vi "Send Launch Models.vi"(8 "error in (no error)":errorcluster, 11 "Message Enqueuer in":refnum<class "Message Enqueuer.lvclass">) -> (0 "error out":errorcluster, 3 "Message Enqueuer out":refnum<class "Message Enqueuer.lvclass">)   [LabVIEW 2015, in "UI Controller.lvlib"]
uses:
  UI Controller.lvlib
  <vilib>/ActorFramework/Message Enqueuer/Message Enqueuer.lvclass
  Models/Settings Model/Settings Model/Settings Model.lvclass
  Models/Message Dialog Model/Message Dialog Model/Message Dialog Model.lvclass
  Models/Print Model/Print Model/Print Model.lvclass
  Hide Subpanel Msg/Hide Subpanel Msg.lvclass
  Hide Subpanel Msg/Hide Subpanel Msg.lvclass/Hide Subpanel Msg.ctl
  <vilib>/ActorFrameworkMVC/Abstract Controller/Abstract Controller Messages/Launch Model Msg/Launch Model Msg.lvclass/Launch Model Msg.ctl
  <vilib>/ActorFramework/Message Enqueuer/Message Enqueuer.lvclass/Message Enqueuer.ctl
  <vilib>/ActorFramework/Self-Addressed Msg/Self-Addressed Msg.lvclass/Self-Addressed Msg.ctl
  Models/Print Model/Print Model/Print Model.lvclass/Print Model.ctl
  <vilib>/ActorFramework/Message Enqueuer/Enqueue.vi
  <vilib>/ActorFramework/Message Priority Queue/Priority Enqueue.vi
  <vilib>/ActorFrameworkMVC/Abstract Controller/Abstract Controller Messages/Launch Model Msg/Launch Model Msg.lvclass
  <vilib>/ActorFramework/Self-Addressed Msg/Self-Addressed Msg.lvclass
panel:
  # "NOTICE -- YOU MUST LEAVE THIS NOTICE IN PLACE.\n\nCopyright (c) 2015, LIANG LIU Shawn.Liu.cn@gmail.com\nAll rights reserved.\n\nRedistribution and use in source and binary forms, with or without modification, are permitted provided that the following conditions are met:\n-Redistributions of source code must retain the above copyright notice, this list of conditions and the following disclaimer.\n-Redistributions in binary form must reproduce the above copyright notice, this list of conditions and the following disclaimer in the documentation and/or other materials provided with the distribution.\n-Neither the name of the eLp nor the names of its contributors may be used to endorse or promote products derived from this software without specific prior written permission.\n\nTHIS SOFTWARE IS PROVIDED BY THE COPYRIGHT HOLDERS AND CONTRIBUTORS \"AS IS\" AND ANY EXPRESS OR IMPLIED WARRANTIES, INCLUDING, BUT NOT LIMITED TO, THE IMPLIED WARRANTIES OF MERCHANTABILITY AND FITNESS FOR A PARTICULAR PURPOSE ARE DISCLAIMED. IN NO EVENT SHALL THE COPYRIGHT HOLDER OR CONTRIBUTORS BE LIABLE FOR ANY DIRECT, INDIRECT, INCIDENTAL, SPECIAL, EXEMPLARY, OR CONSEQUENTIAL DAMAGES (INCLUDING, BUT NOT LIMITED TO, PROCUREMENT OF SUBSTITUTE GOODS OR SERVICES; LOSS OF USE, DATA, OR PROFITS; OR BUSINESS INTERRUPTION) HOWEVER CAUSED AND ON ANY THEORY OF LIABILITY, WHETHER IN CONTRACT, STRICT LIABILITY, OR TORT (INCLUDING NEGLIGENCE OR OTHERWISE) ARISING IN ANY WAY OUT OF THE USE OF THIS SOFTWARE, EVEN IF ADVISED OF THE POSSIBILITY OF SUCH DAMAGE."
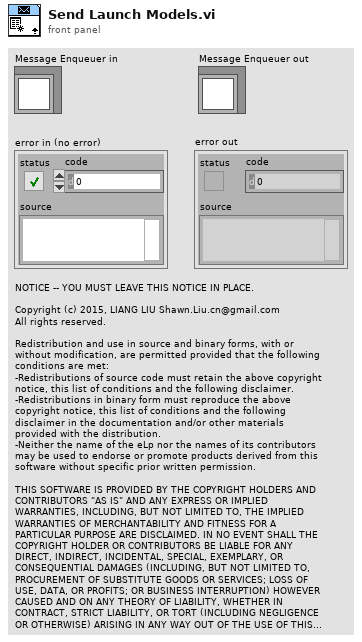
[diagram p1: front panel]
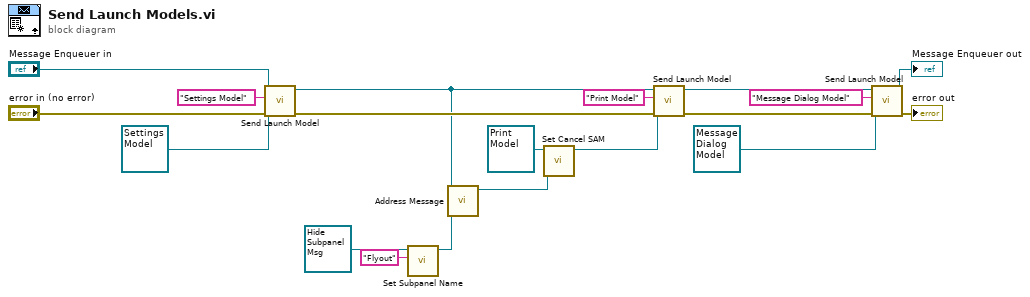
[diagram p0: block diagram]
diagram:
  n1 = call <vilib>:"Send Launch Model.vi"("error in (no error)"="error in (no error)", "Model"=refnum<class "Settings Model.lvclass"> refnum ("Settings Model.lvlib:Settings Model.lvclass"), "Model Name"="Settings Model", "Message Enqueuer"="Message Enqueuer in") -> ("error out"=w12:errorcluster, "Message Enqueuer out"=w3:refnum<class "Message Enqueuer.lvclass">)  [unwired: 6 in]
  n2 = call "Set Subpanel Name.vi"("Subpanel Name"="Flyout", "Hide Subpanel Msg in"=refnum<class "Hide Subpanel Msg.lvclass"> refnum ("View Controller.lvlib:Move Subpanel Msg.lvclass")) -> ("Hide Subpanel Msg out"=w4:refnum<class "Hide Subpanel Msg.lvclass">)  [unwired: 9 in]
  n3 = call <vilib>:"Address Message.vi"("Message"=w4, "Destination"=w3) -> ("Self-Addressed Message"=w2:refnum<class "Self-Addressed Msg.lvclass">)  [unwired: 9 in]
  n4 = call "Set Cancel SAM.vi"("Cancel SAM"=w2, "Print Model in"=refnum<class "Print Model.lvclass"> refnum ("Print Model.lvlib:Print Model.lvclass")) -> ("Print Model out"=w6:refnum<class "Print Model.lvclass">)  [unwired: 9 in]
  n5 = call <vilib>:"Send Launch Model.vi"("error in (no error)"=w12, "Model"=w6, "Model Name"="Print Model", "Message Enqueuer"=w3) -> ("error out"=w11:errorcluster, "Message Enqueuer out"=w10:refnum<class "Message Enqueuer.lvclass">)  [unwired: 6 in]
  n6 = call <vilib>:"Send Launch Model.vi"("error in (no error)"=w11, "Model"=refnum<class "Message Dialog Model.lvclass"> refnum ("Message Model.lvlib:Message Model.lvclass"), "Model Name"="Message Dialog Model", "Message Enqueuer"=w10) -> ("error out"=→"error out":errorcluster, "Message Enqueuer out"=→"Message Enqueuer out":refnum<class "Message Enqueuer.lvclass">)  [unwired: 6 in]
